vi "niRFUtil ERR Check Valid Input (I32).vi"(0 "Property Value":i32, 1 "Property Name":string, 7 "Upper Limit":i32=2147483647, 9 "Lower Limit":i32=-2147483648, 11 "error in (no error)":errorcluster, 12 "Error Code":i32=-379001) -> (15 "error out":errorcluster)   [LabVIEW 2015, in "niRFUtil.lvlib"]
uses:
  niRFUtil.lvlib
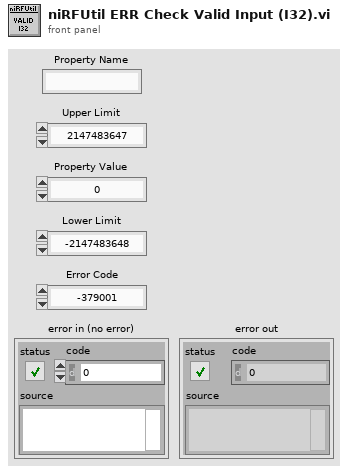
[diagram p1: front panel]
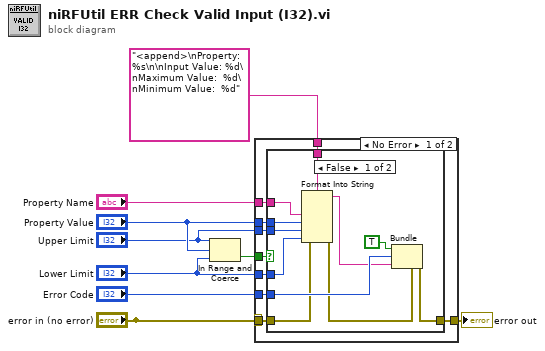
[diagram p0: block diagram]
diagram:
  n1 = In Range and Coerce(upper limit="Upper Limit", x="Property Value", lower limit="Lower Limit") -> (In Range?=w3:bool)  [unwired: 1 out]
  n2 = case shown="No Error" "error in (no error)" {
    tunnel: "<append>\nProperty: %s\n\nInput Value: %d\nMaximum Value:  %d\nMinimum Value:  %d" ("initial string") -> [w18 _]
    tunnel: "Property Value" -> [w17 _]
    tunnel: "Upper Limit" -> [w16 _]
    tunnel: "Lower Limit" -> [w15 _]
    tunnel: "Property Name" -> [w14 _]
    tunnel: "Error Code" -> [w13 _]
    tunnel: w3 -> [w12 _]
    tunnel: "error in (no error)" -> [w11 w31]
    tunnel: [w10 w31] -> w2
    frame No Error {
      n3 = case shown="False" w12 {
        tunnel: w18 -> [w29 _]
        tunnel: w17 -> [w28 _]
        tunnel: w16 -> [w27 _]
        tunnel: w15 -> [w26 _]
        tunnel: w14 -> [w25 _]
        tunnel: w13 -> [w23 _]
        tunnel: w11 -> [w20 w30]
        tunnel: [w21 w30] -> w10
        frame False {
          n4 = Format Into String(format string=w29, error in=w20, w25, w28, w27, w26) -> (resulting string=w22:string, error out=w19:errorcluster)  [unwired: 1 in]
          n5 = Bundle(cluster=w19, "status"=TRUE ("show call chain? (False)"), "code"=w23, "source"=w22) -> (w21:errorcluster)
        }
        frame True {
        }
      }
    }
    frame Error {
    }
  }
  "error out" <- w2
